vi "Personlist.vi"() -> ()   [LabVIEW 2020]
uses:
  PL_Global.vi
panel:
  in  "stop":bool
  in  "PERSON LIST":cluster{"NAMES":string[], "ID":dbl[]}
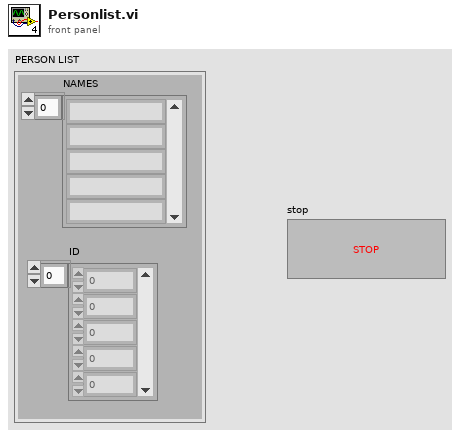
[diagram p1: front panel]
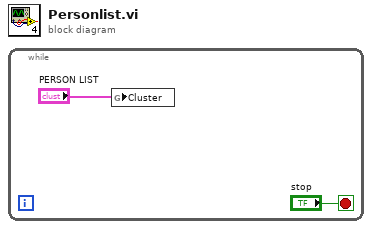
[diagram p0: block diagram]
diagram:
  n1 = while {
    stop <- "stop" stop-if-true
    n2 = global write "PL_Global.vi" "Cluster"("PERSON LIST") -> ()
  }
